vi "licz_piq - Kopia.vi"(7 "x":dbl, 8 "b":dbl, 9 "a":dbl, 10 "delta":dbl) -> (1 "Postać kanoniczna":string, 2 "q":dbl, 3 "p":dbl)   [LabVIEW 2020]
doc: "obliczanie p i q"
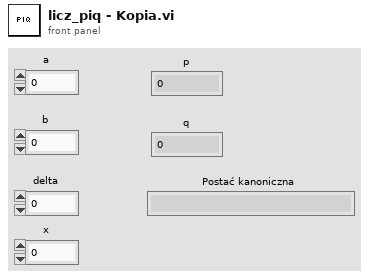
[diagram p1: front panel]
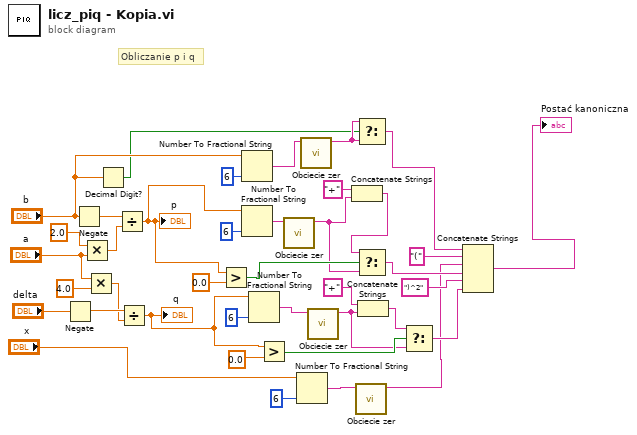
[diagram p0: block diagram]
diagram:
  # "Obliczanie p i q"
  n1 = Negate(x="delta") -> (-x=w35:dbl)
  n2 = Negate(x="b") -> (-x=w39:dbl)
  n3 = Multiply(x=2.0, y="a") -> (x*y=w38:dbl)
  n4 = Multiply(x="a", y=4.0) -> (x*y=w34:dbl)
  n5 = Decimal Digit?(1:"b") -> (0:w5:bool)
  n6 = Divide(x=w39, y=w38) -> (x/y=w3:dbl)
  "p" <- w3
  n7 = Divide(x=w35, y=w34) -> (x/y=w2:dbl)
  "q" <- w2
  n8 = Greater?(x=w3, y=0.0) -> (0:w18:bool)
  n9 = Number To Fractional String(number="b", precision (6)=i16 6) -> (F-format string=w13:string)  [unwired: 2 in]
  n10 = Number To Fractional String(number=w3, precision (6)=i16 6) -> (F-format string=w11:string)  [unwired: 2 in]
  n11 = Number To Fractional String(number=w2, precision (6)=i16 6) -> (F-format string=w9:string)  [unwired: 2 in]
  n12 = Greater?(x=w2, y=0.0) -> (0:w19:bool)
  n13 = call "Obciecie zer.vi"("Wejściowa liczba"=w11) -> ("Wyjściowa liczba"=w10:string)  [unwired: 10 in]
  n14 = Number To Fractional String(number="x", precision (6)=i16 6) -> (F-format string=w15:string)  [unwired: 2 in]
  n15 = call "Obciecie zer.vi"("Wejściowa liczba"=w13) -> ("Wyjściowa liczba"=w12:string)  [unwired: 10 in]
  n16 = call "Obciecie zer.vi"("Wejściowa liczba"=w9) -> ("Wyjściowa liczba"=w8:string)  [unwired: 10 in]
  n17 = Concatenate Strings("+" ("string"), w10) -> (w27:string)
  n18 = call "Obciecie zer.vi"("Wejściowa liczba"=w15) -> ("Wyjściowa liczba"=w14:string)  [unwired: 10 in]
  n19 = Select(t=w12, s=w5, f=w12) -> (s? t:f=w17:string)
  n20 = Select(t=w27, s=w18, f=w10) -> (s? t:f=w26:string)
  n21 = Concatenate Strings("+" ("string"), w8) -> (w22:string)
  n22 = Select(t=w22, s=w19, f=w8) -> (s? t:f=w21:string)
  n23 = Concatenate Strings(w17, "(" ("string"), w14, w26, ")^2" ("string"), w21) -> (→"Postać kanoniczna":string)
